vi "Array of Objects to JSON Array.vi"(8 "error in (no error)":errorcluster, 11 "Array of JSON":string[](array[string])) -> (0 "error out":errorcluster, 3 "JSON Array":string)   [LabVIEW 2019, in "JSON-RPC.lvclass"]
uses:
  JSON-RPC.lvclass
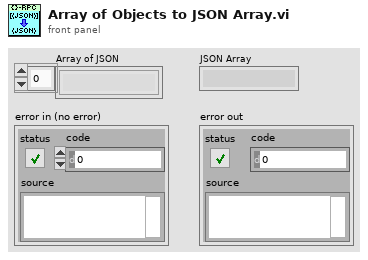
[diagram p1: front panel]
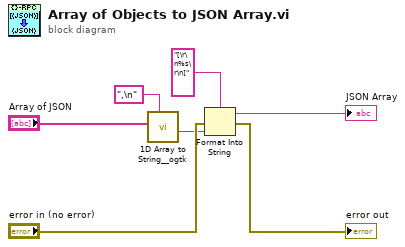
[diagram p0: block diagram]
diagram:
  n1 = call "1D Array to String__ogtk.vi"("delimiter (Tab)"=",\n", "Array of Strings"="Array of JSON") -> ("delimited string"=w5:string)  [unwired: 9 in]
  n2 = Format Into String(format string="[\r\n%s\r\n]", error in="error in (no error)", w5) -> (resulting string=→"JSON Array":string, error out=→"error out":errorcluster)  [unwired: 1 in]
